vi "Next Step.vi"(8 "error in (no error)":errorcluster, 11 "Pulse Gen Basic Scan in":refnum<class "Pulse Gen Basic Scan.lvclass">) -> (0 "error out":errorcluster, 1 "Current Step":u32, 2 "Current Position":dbl, 3 "Pulse Gen Basic Scan out":refnum<class "Pulse Gen Basic Scan.lvclass">)   [LabVIEW 2009, in "Pulse Gen Basic Scan.lvclass"]
doc: "(Dynamic) Move to the next preconfigured step of this Scanner, and return the current position (actual, not intended) of this Scanner. Increment the step counter by one."
uses:
  Pulse Gen Basic Scan.lvclass
  Scanner/Scanner.lvclass
  Pulse Gen Basic Scan.lvclass/Pulse Gen Basic Scan.ctl
  Instruments/Utility Classes/Scannable/Scannable.lvclass
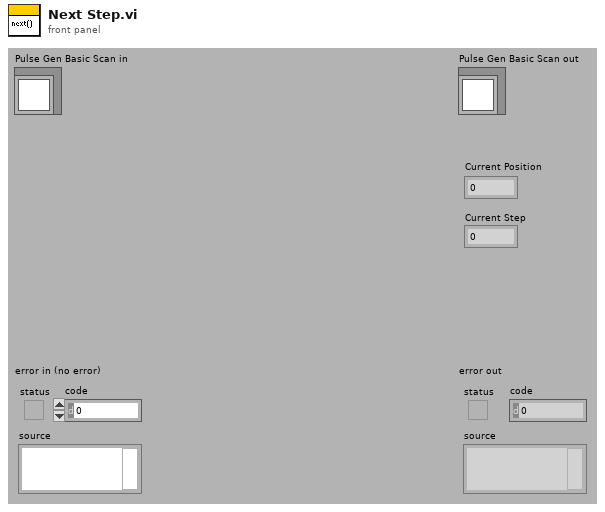
[diagram p1: front panel]
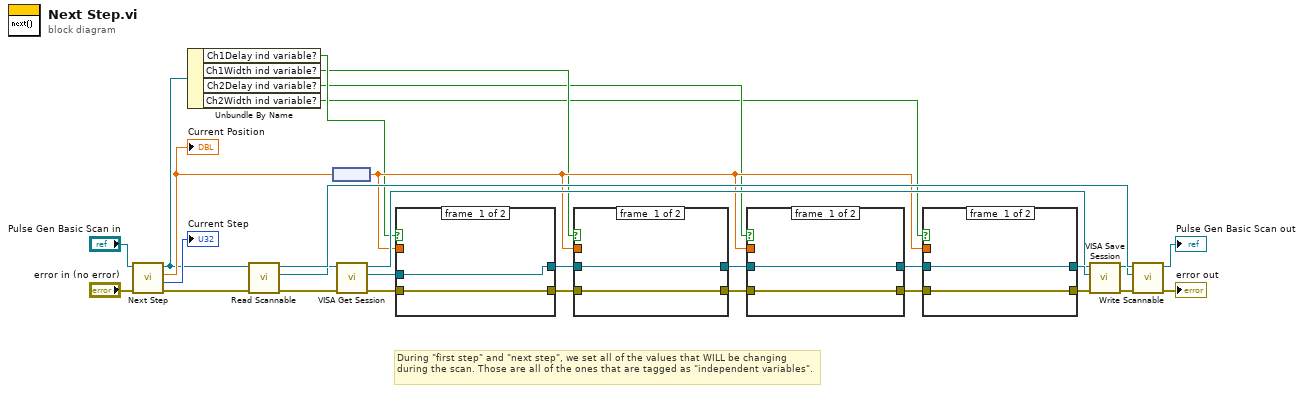
[diagram p0: block diagram]
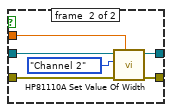
[diagram p2: hidden frame]
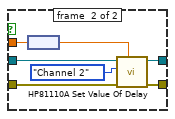
[diagram p3: hidden frame]
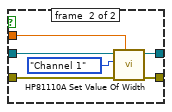
[diagram p4: hidden frame]
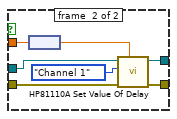
[diagram p5: hidden frame]
diagram:
  # "During \"first step\" and \"next step\", we set all of the values that WILL be changing during the scan. Those are all of the ones that are tagged as \"independent variables\"."
  n1 = call-parent "Next Step.vi"("error in (no error)"="error in (no error)", "Scanner in"="Pulse Gen Basic Scan in") -> ("error out"=w1:errorcluster, "Current Step"=→"Current Step":u32, "Current Position"=w5:dbl, "Scanner out"=w4:refnum<class "Pulse Gen Basic Scan.lvclass">)  [unwired: 6 in]
  "Current Position" <- w5
  n2 = Unbundle By Name(w4) -> ("Ch1Delay ind variable?"=w9:bool, "Ch1Width ind variable?"=w8:bool, "Ch2Delay ind variable?"=w7:bool, "Ch2Width ind variable?"=w6:bool)
  n3 = call-dynamic "Read Scannable.vi"("error in (no error)"=w1, "Scanner.lvclass in"=w4) -> ("error out"=w19:errorcluster, "Scannable.lvclass"=w16:refnum<class "Scannable.lvclass">, "Scanner.lvclass out"=w20:refnum<class "Pulse Gen Basic Scan.lvclass">)  [unwired: 7 out]
  n4 = node(w5) -> (w11:dbl[unit])
  n5 = call-dynamic "VISA Get Session.vi"("error in (no error)"=w19, "Instrument.lvclass in"=w16) -> ("error out"=w18:errorcluster, "VISA Resource Name"=w10:refnum<visa-resource-name>, "Instrument.lvclass out"=w15:refnum<class "Scannable.lvclass">)  [unwired: 7 out]
  n6 = case shown="True" w9 {
    tunnel: [w30 w38] -> w26
    tunnel: w18 -> [w31 w37]
    tunnel: [w31 w36] -> w23
    tunnel: w11 -> [_ w34]
    tunnel: w10 -> [w30 w32]
    frame #0 {
    }
    frame #1 {
      n7 = node(w34) -> (w33:dbl)
      n8 = call "HP81110A Set Value Of Delay.vi"("Delay Value (0.0)"=w33, "error in (no error)"=w37, "Channel (1:Channel 1)"=enum16{"Channel All ", "Channel 1", "Channel 2"}."Channel 1", "VISA session"=w32) -> ("error out"=w36:errorcluster, "dup VISA session"=w38:refnum<visa-resource-name>)  [unwired: 6 in]
    }
  }
  n9 = case shown="True" w8 {
    tunnel: w26 -> [w40 w46]
    tunnel: [w40 w45] -> w25
    tunnel: w23 -> [w39 w44]
    tunnel: [w39 w43] -> w22
    tunnel: w11 -> [_ w41]
    frame #0 {
    }
    frame #1 {
      n10 = call "HP81110A Set Value Of Width.vi"("Width Value (100.0E-9)"=w41, "error in (no error)"=w44, "Channel (1:Channel 1)"=enum16{"Channel All ", "Channel 1", "Channel 2"}."Channel 1", "VISA session"=w46) -> ("error out"=w43:errorcluster, "dup VISA session"=w45:refnum<visa-resource-name>)  [unwired: 6 in]
    }
  }
  n11 = case shown="True" w7 {
    tunnel: w25 -> [w48 w55]
    tunnel: [w48 w54] -> w24
    tunnel: w22 -> [w47 w53]
    tunnel: [w47 w52] -> w21
    tunnel: w11 -> [_ w50]
    frame #0 {
    }
    frame #1 {
      n12 = node(w50) -> (w49:dbl)
      n13 = call "HP81110A Set Value Of Delay.vi"("Delay Value (0.0)"=w49, "error in (no error)"=w53, "Channel (1:Channel 1)"=enum16{"Channel All ", "Channel 1", "Channel 2"}."Channel 2", "VISA session"=w55) -> ("error out"=w52:errorcluster, "dup VISA session"=w54:refnum<visa-resource-name>)  [unwired: 6 in]
    }
  }
  n14 = case shown="True" w6 {
    tunnel: w24 -> [w56 w63]
    tunnel: w21 -> [w57 w62]
    tunnel: [w57 w61] -> w13
    tunnel: w11 -> [_ w59]
    tunnel: [w56 w58] -> w17
    frame #0 {
    }
    frame #1 {
      n15 = call "HP81110A Set Value Of Width.vi"("Width Value (100.0E-9)"=w59, "error in (no error)"=w62, "Channel (1:Channel 1)"=enum16{"Channel All ", "Channel 1", "Channel 2"}."Channel 2", "VISA session"=w63) -> ("error out"=w61:errorcluster, "dup VISA session"=w58:refnum<visa-resource-name>)  [unwired: 6 in]
    }
  }
  n16 = call-dynamic "VISA Save Session.vi"("error in (no error)"=w13, "VISA Resource Name"=w17, "Instrument.lvclass in"=w15) -> ("error out"=w12:errorcluster, "Instrument.lvclass out"=w14:refnum<class "Scannable.lvclass">)  [unwired: 7 out]
  n17 = call-dynamic "Write Scannable.vi"("error in (no error)"=w12, "Scannable.lvclass"=w14, "Scanner.lvclass in"=w20) -> ("error out"=→"error out":errorcluster, "Scanner.lvclass out"=→"Pulse Gen Basic Scan out":refnum<class "Pulse Gen Basic Scan.lvclass">)  [unwired: 7 out]
